vi "Delete.vi"(8 "error in (no error)":errorcluster, 11 "Service in":refnum<class "Service.lvclass">) -> (0 "error out":errorcluster)   [LabVIEW 2024, in "Ramses Framework.lvlib" / "Service.lvclass"]
uses:
  Service.lvclass
  Service.lvclass/Service.ctl
  Communications/Server/Base Server/Server.lvclass
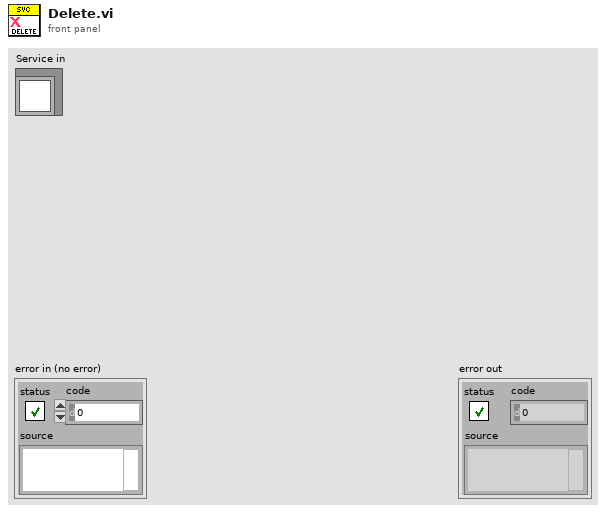
[diagram p1: front panel]
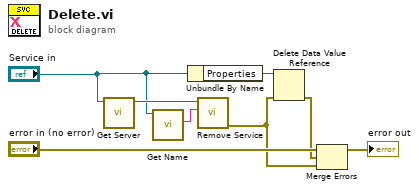
[diagram p0: block diagram]
diagram:
  n1 = call "Get Server.vi"("Service in"="Service in") -> ("Server"=w4:refnum<class "Server.lvclass">)  [unwired: 9 in, 1 out]
  n2 = call "Get Name.vi"("Service in"="Service in") -> ("Name"=w2:string)  [unwired: 8 in, 2 out]
  n3 = Unbundle By Name("Service in") -> ("Properties"=w8:refnum<data-value>)
  n4 = call-dynamic "Remove Service.vi"("Class Name"=w2, "Server in"=w4) -> ("error out"=w1:errorcluster)  [unwired: 8 in, 1 out]
  n5 = Delete Data Value Reference(data value reference=w8, error in=w1) -> (error out=w5:errorcluster)  [unwired: 1 out]
  n6 = Merge Errors("error in (no error)", w5, w1) -> (→"error out":errorcluster)
